vi "ChangeWhileMeasuring.vi"(8 "error in (no error)":errorcluster, 11 "NHRGridSim in":refnum<class "NHRGridSim.lvclass">) -> (0 "error out":errorcluster, 1 "InstrumentSettings":bool, 2 "OutputOrLoadValue":bool, 3 "NHRGridSim out":refnum<class "NHRGridSim.lvclass">)   [LabVIEW 2018, in "AcPwrPlugins.lvlib" / "NHRGridSim.lvclass"]
doc: "This VI reads the instrument property ChangeWhileMeasuring to see if the instrument can change the value of a property (voltage, current, etc) while the device is simultaneously aquiring measurements."
uses:
  NHRGridSim.lvclass
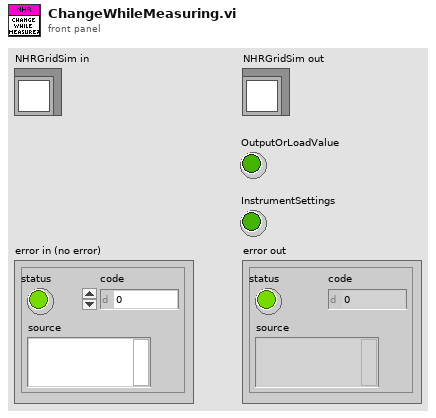
[diagram p1: front panel]
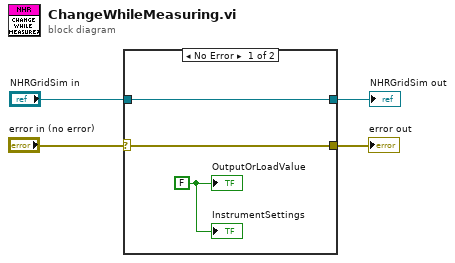
[diagram p0: block diagram]
diagram:
  n1 = case shown="No Error" "error in (no error)" {
    selector: "error in (no error)" -> [w7 w9]
    tunnel: [w7 w9] -> w1
    tunnel: "NHRGridSim in" -> [w6 w8]
    tunnel: [w6 w8] -> w2
    frame No Error {
      w5 = FALSE ("OutputOrLoadValue")
      "InstrumentSettings" <- w5
      "OutputOrLoadValue" <- w5
    }
    frame Error {
    }
  }
  "error out" <- w1
  "NHRGridSim out" <- w2
